vi "Init.vi"(8 "error in (no error)":errorcluster, 11 "Channel Info":T1) -> (0 "error out":errorcluster, 3 "Channel Config out":refnum<class "Channel Config.lvclass">)   [LabVIEW 2020, in "Vecto.lvlib" / "Channel Config.lvclass"]
uses:
  Channel Config.lvclass
  Channel Info.ctl
  Channel Config.lvclass/Channel Config.ctl
  Vecto.lvlib
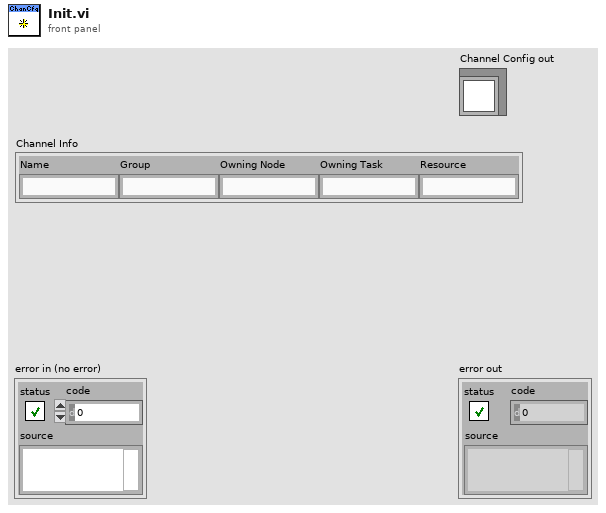
[diagram p1: front panel]
types:
  T1 = typedef "Vecto.lvlib/Channel Info.ctl" = cluster{"Name":string, "Group":string, "Owning Node":string, "Owning Task":string, "Resource":string}
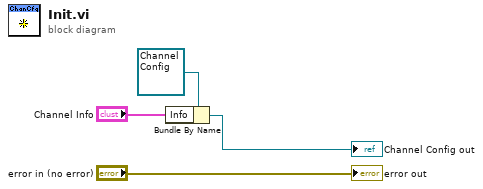
[diagram p0: block diagram]
diagram:
  n1 = Bundle By Name(cluster=refnum<class "Channel Config.lvclass"> refnum ("Channel Config in"), "Info"="Channel Info") -> (→"Channel Config out":refnum<class "Channel Config.lvclass">)
  "error out" <- "error in (no error)"
